vi "数据表-删除数据.vi"(4 "元素名[]-探测器列表":string[](array[string]), 5 "表名-设备表":string, 6 "元素名[]-累积记录":string[](array[string]), 8 "error in (no error)":errorcluster, 10 "要删除的记录":T1, 11 "数据库引用":T3) -> (0 "error out":errorcluster, 2 "删除量":dbl, 3 "connection reference out":T3)   [LabVIEW 2017]
doc: "删除部分数据时候, 返回删除量为有效值,\n删除全部数据(清零操作), 返回删除量为 正无穷."
uses:
  <vilib>/addons/database/Connection.llb/Conn ObjectReference.ctl
  <vilib>/addons/database/NI_Database_API.lvlib
panel:
  out "Result":string caption="sql-累积剂量变更"
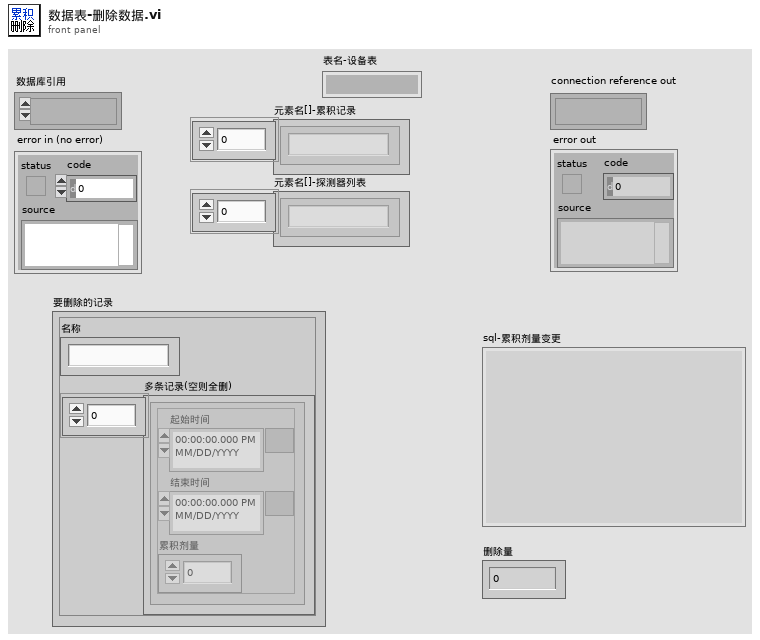
[diagram p1: front panel]
types:
  T1 = typedef "删除记录输入.ctl" = cluster{"名称":string, "多条记录(空则全删)":T2[]}
  T2 = typedef "单条累积记录.ctl" = cluster{"起始时间":timestamp, "结束时间":timestamp, "累积剂量":dbl}
  T3 = typedef "NI_Database_API.lvlib/Conn ObjectReference.ctl" = refnum<k1>
  T4 = typedef "探测器信息.ctl" = cluster{"网络地址":string, "名称":string, "备注":string, "累积剂量":dbl, "累积限值":dbl, "硬件剂量率限值":T5, "剂量率限值1":dbl, "剂量率限值2":dbl, "报警方式":T6}
  T5 = typedef "探头剂量率限值选择.ctl" = enum16{"一级限值", "二级限值"}
  T6 = typedef "报警方式选择.ctl" = enum16{"常报警", "自动静音", "手动静音"}
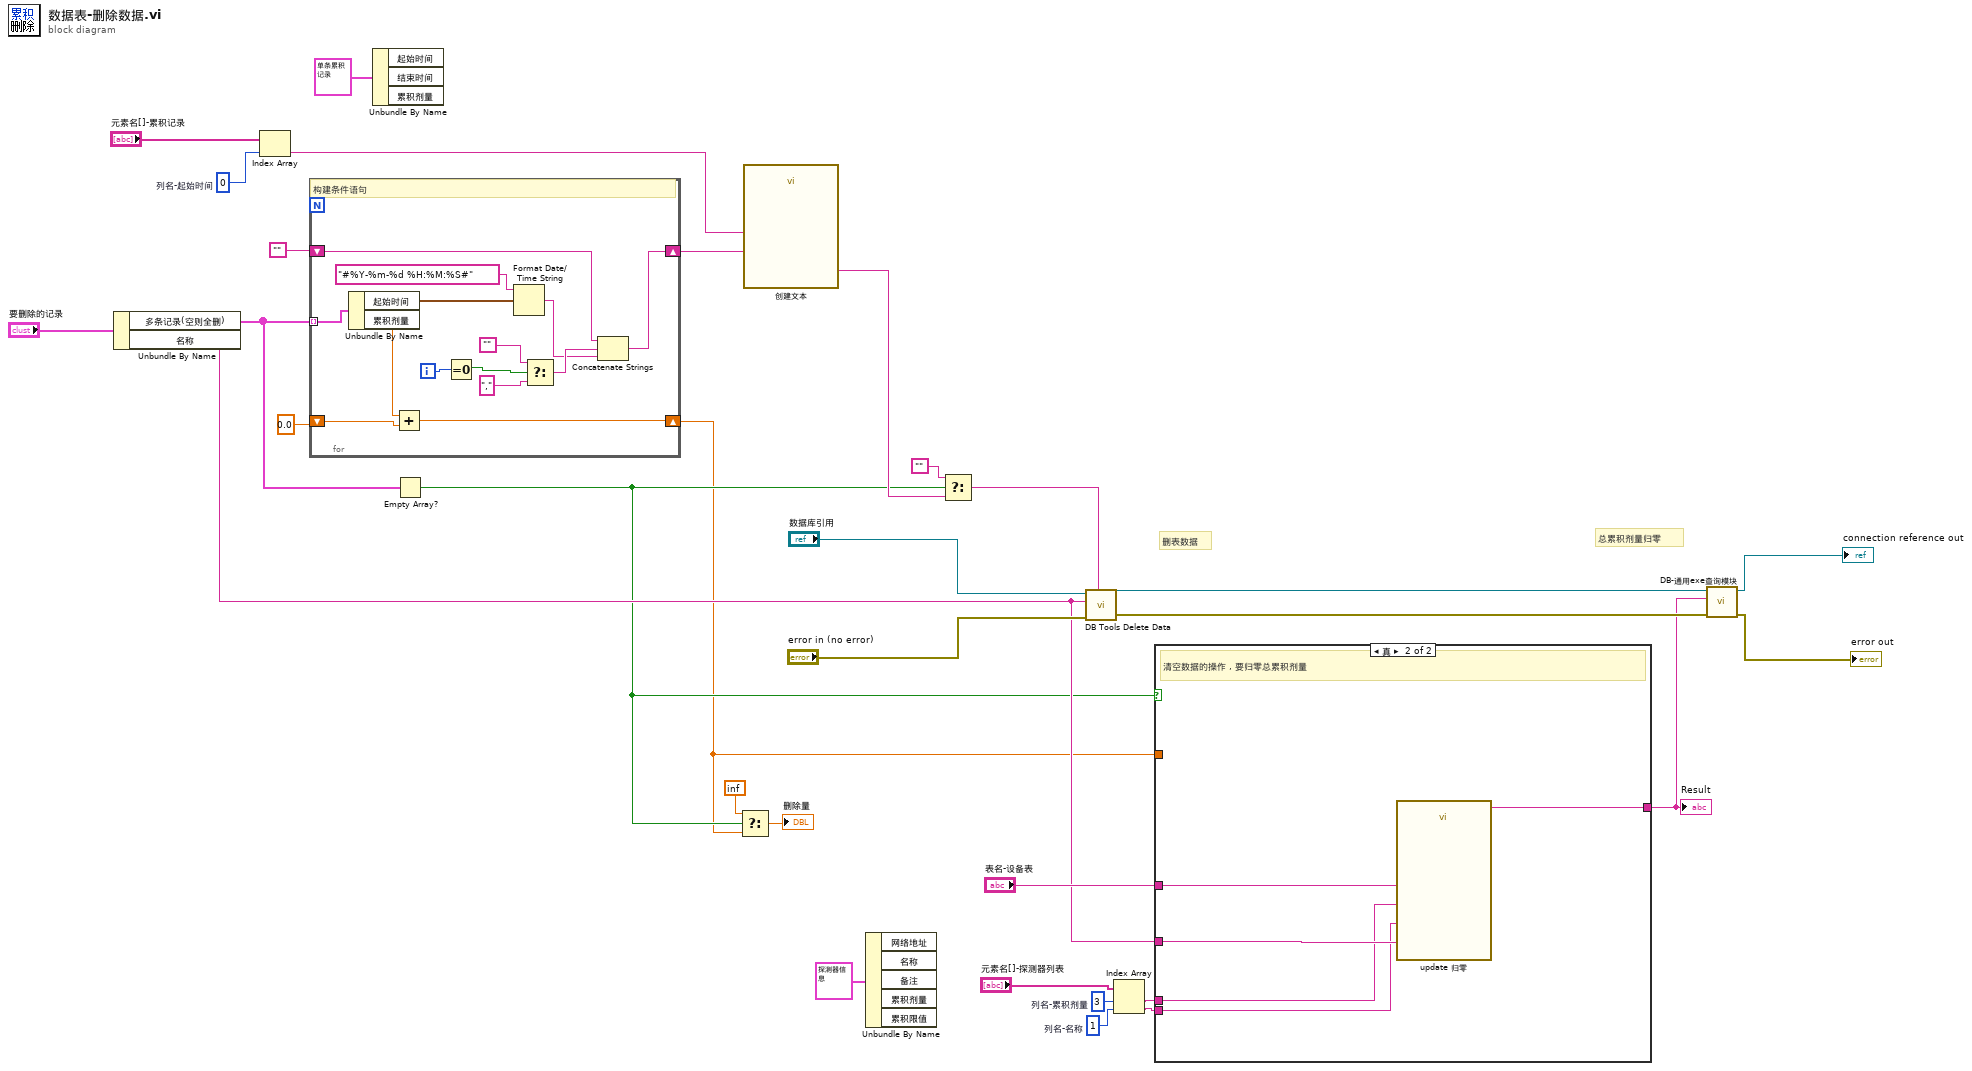
[diagram p0: block diagram]
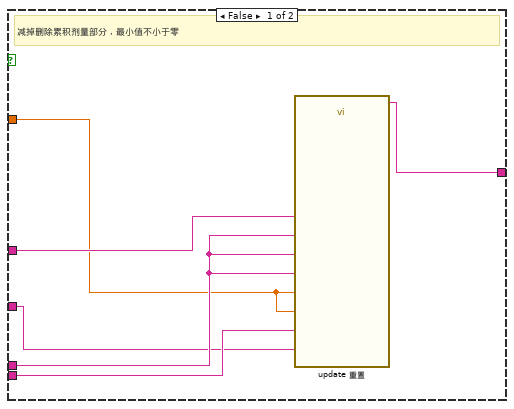
[diagram p2: hidden frame]
diagram:
  w15 = 1  # 列名-名称
  w14 = 3  # 列名-累积剂量
  w28 = 0  # 列名-起始时间
  # "总累积剂量归零"
  # "删表数据"
  n1 = Unbundle By Name("要删除的记录") -> ("多条记录(空则全删)"=w6:T2[], "名称"=w5:string)
  n2 = Index Array(array="元素名[]-累积记录", index=w28) -> (element=w26:string)
  n3 = for {
    tunnel: w6 -> [w45] mode=indexing
    shift-right: [w35] -> w25
    shift-left: "" -> [w36]
    shift-right: [w32] -> w2
    shift-left: 0.0 ("累积剂量") -> [w34]
    i -> [w44]
    # "构建条件语句"
    n4 = Unbundle By Name(w45) -> ("起始时间"=w43:timestamp, "累积剂量"=w33:dbl)
    n5 = Add(x=w33, y=w34) -> (x+y=w32:dbl)
    n6 = Equal To 0?(x=w44) -> (x = 0?=w41:bool)
    n7 = Format Date/Time String(time format string (%c)="#%Y-%m-%d %H:%M:%S#" ("时间格式字符串(%c)"), seconds (now)=w43) -> (date/time string=w37:string)  [unwired: 1 in]
    n8 = Select(t="", s=w41, f="," ("字符串")) -> (s? t:f=w38:string)
    n9 = Concatenate Strings(w36, w38, w37) -> (w35:string)
  }
  n10 = Unbundle By Name(T2 {"起始时间"=timestamp(0 s since 1904-01-01), "结束时间"=timestamp(0 s since 1904-01-01), "累积剂量"=0.0} ("累积记录")) -> ()  [unwired: 3 out]
  n11 = Empty Array?(array=w6) -> (empty?=w4:bool)
  n12 = Select(t=inf, s=w4, f=w2) -> (s? t:f=→"删除量":dbl)
  n13 = call "创建文本"("列名-起始时间"=w26, "时间集合"=w25) -> ("Result"=w22:string)  [unwired: 12 in, 1 out]
  n14 = Unbundle By Name(T4 {"网络地址"="", "名称"="", "备注"="", "累积剂量"=0.0, "累积限值"=0.0, "硬件剂量率限值"=enum."一级限值", "剂量率限值1"=0.0, "剂量率限值2"=0.0, "报警方式"=enum."常报警"} ("探测器信息")) -> ()  [unwired: 5 out]
  n15 = Select(t="", s=w4, f=w22) -> (s? t:f=w21:string)
  n16 = call <vilib>:"DB Tools Delete Data.vi"("condition"=w21, "error in (no error)"="error in (no error)", "table"=w5, "connection reference"="数据库引用") -> ("error out"=w17:errorcluster, "connection reference out"=w18:T3)  [unwired: 6 in]
  n17 = Index Array(array="元素名[]-探测器列表", index #1=w14, index #2=w15) -> (element #1=w11:string, element #2=w10:string)
  n18 = case shown="真" w4 {
    tunnel: w5 -> [w47 w56]
    tunnel: [w46 w55] -> w8
    tunnel: "表名-设备表" -> [w51 w54]
    tunnel: w11 -> [w50 w53]
    tunnel: w10 -> [w48 w52]
    tunnel: w2 -> [w49 _]
    frame False {
      # "减掉删除累积剂量部分 , 最小值不小于零"
      n19 = call "update 重置"("删除量"=w49, "删除量1"=w49, "探测器名称"=w47, "表名-设备表"=w51, "列名-累积剂量"=w50, "列名-累积剂量1"=w50, "列名-累积剂量2"=w50, "列名-名称"=w48) -> ("Result"=w46:string)  [unwired: 6 in, 1 out]
    }
    frame True {
      # "清空数据的操作 , 要归零总累积剂量"
      n20 = call "update 归零"("探测器名称"=w56, "表名-设备表"=w54, "列名-累积剂量"=w53, "列名-名称"=w52) -> ("Result"=w55:string)  [unwired: 10 in, 1 out]
    }
  }
  "Result" <- w8
  n21 = call "DB-通用exe查询模块.vi"("error in (no error)"=w17, "SQL query"=w8, "数据库连接引用"=w18) -> ("error out"=→"error out":errorcluster, "数据库连接引用out"=→"connection reference out":T3)  [unwired: 4 in, 3 out]
